vi "AlliGator Format Path String for Python.vi"(8 "Error In":errorcluster, 11 "Python Plugin Dialog Output":string[][](array[string])) -> (0 "Error Out":errorcluster, 3 "Python Plugin Dialog Output":string[][](array[string]))   [LabVIEW 2021, in "AlliGator Python Plugins.lvlib"]
doc: "Formats path for python function consumption."
uses:
  AlliGator Python Plugins.lvlib
panel:
  # "see the AlliGator License on the block diagram (Ctrl+E or Window:Show Block Diagram)"
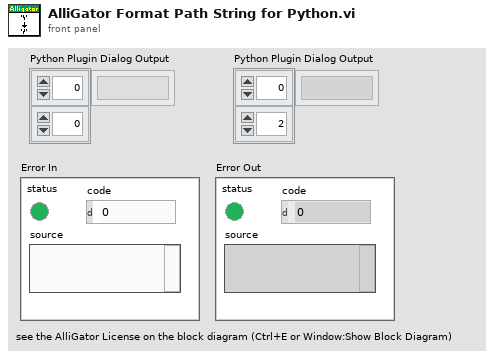
[diagram p1: front panel]
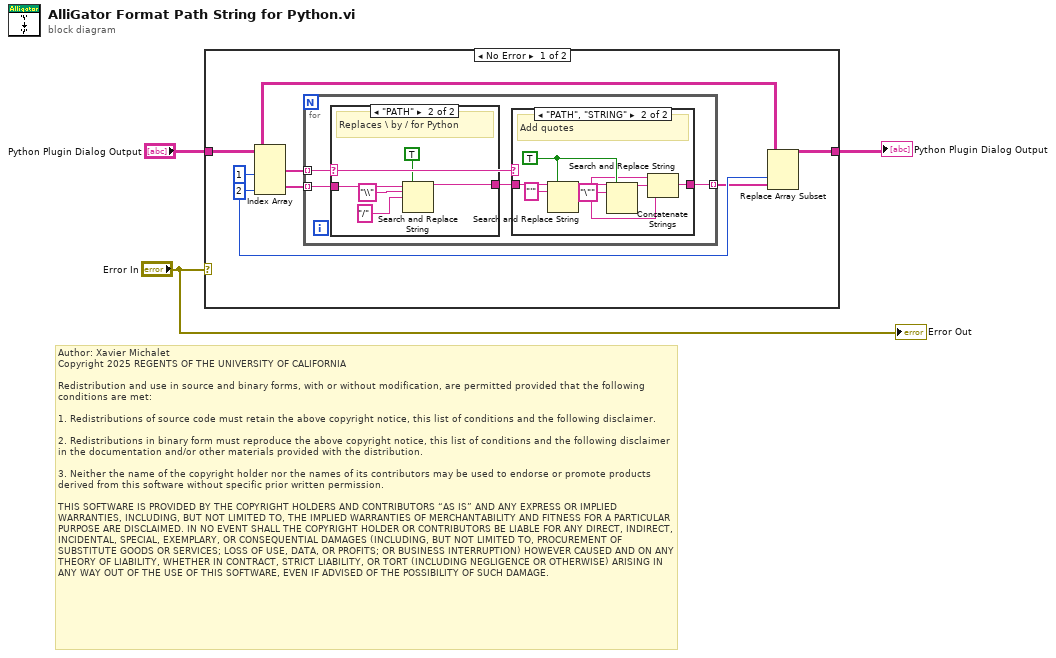
[diagram p0: block diagram]
diagram:
  # "Author: Xavier Michalet\nCopyright 2025 REGENTS OF THE UNIVERSITY OF CALIFORNIA\n\nRedistribution and use in source and binary forms, with or without modification, are permitted provided that the following conditions are met:\n\n1. Redistributions of source code must retain the above copyright notice, this list of conditions and the following disclaimer.\n\n2. Redistributions in binary form must reproduce the above copyright notice, this list of conditions and the following disclaimer in the documentation and/or other materials provided with the distribution.\n\n3. Neither the name of the copyright holder nor the names of its contributors may be used to endorse or promote products derived from this software without specific prior written permission.\n\nTHIS SOFTWARE IS PROVIDED BY THE COPYRIGHT HOLDERS AND CONTRIBUTORS “AS IS” AND ANY EXPRESS OR IMPLIED WARRANTIES, INCLUDING, BUT NOT LIMITED TO, THE IMPLIED WARRANTIES OF MERCHANTABILITY AND FITNESS FOR A PARTICULAR PURPOSE ARE DISCLAIMED. IN NO EVENT SHALL THE COPYRIGHT HOLDER OR CONTRIBUTORS BE LIABLE FOR ANY DIRECT, INDIRECT, INCIDENTAL, SPECIAL, EXEMPLARY, OR CONSEQUENTIAL DAMAGES (INCLUDING, BUT NOT LIMITED TO, PROCUREMENT OF SUBSTITUTE GOODS OR SERVICES; LOSS OF USE, DATA, OR PROFITS; OR BUSINESS INTERRUPTION) HOWEVER CAUSED AND ON ANY THEORY OF LIABILITY, WHETHER IN CONTRACT, STRICT LIABILITY, OR TORT (INCLUDING NEGLIGENCE OR OTHERWISE) ARISING IN ANY WAY OUT OF THE USE OF THIS SOFTWARE, EVEN IF ADVISED OF THE POSSIBILITY OF SUCH DAMAGE."
  n1 = case shown="No Error" "Error In" {
    tunnel: "Python Plugin Dialog Output" -> [w10 w29]
    tunnel: [w9 w29] -> w1
    frame No Error {
      w5 = 2 ("disabled index (col)")
      n2 = Index Array(array=w10, index (col) #1=1 ("disabled index (col)"), index (col) #2=w5) -> (element #1=w7:string[], element #2=w6:string[])  [unwired: 2 in]
      n3 = for {
        tunnel: w7 -> [w13] mode=indexing
        tunnel: w6 -> [w14] mode=indexing
        tunnel: [w11] -> w4 mode=indexing
        n4 = case shown="\"PATH\"" w13 {
          tunnel: w14 -> [w23 w28]
          tunnel: [w23 w24] -> w12
          frame Default {
          }
          frame "PATH" {
            # "Replaces \\ by / for Python"
            n5 = Search and Replace String(replace all?=TRUE ("replace all? (F)"), input string=w28, search string="\\", replace string="/" ("replace string (\"\")")) -> (result string=w24:string)  [unwired: 4 in, 3 out]
          }
        }
        n6 = case shown="\"PATH\", \"STRING\"" w13 {
          tunnel: w12 -> [w15 w22]
          tunnel: [w15 w16] -> w11
          frame Default {
          }
          frame "PATH", "STRING" {
            w17 = "\"" ("search string")
            w19 = TRUE ("replace all? (F)")
            # "Add quotes"
            n7 = Search and Replace String(replace all?=w19, input string=w22, search string="'") -> (result string=w20:string)  [unwired: 5 in, 3 out]
            n8 = Search and Replace String(replace all?=w19, input string=w20, search string=w17) -> (result string=w18:string)  [unwired: 5 in, 3 out]
            n9 = Concatenate Strings(w17, w18, w17) -> (w16:string)
          }
        }
      }
      n10 = Replace Array Subset(array=w10, new element=w4, index (col)=w5) -> (w9:string[][])  [unwired: 1 in]
    }
    frame Error {
    }
  }
  "Python Plugin Dialog Output" <- w1
  "Error Out" <- "Error In"
